vi "number to Boolean.vi"(1 "Numeric":dbl) -> (0 "Boolean":bool)   [LabVIEW 2023]
doc: "If input number (real or integer) is zero, outputs a \"false\". Otherwise, outputs a \"true\"."
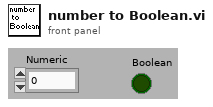
[diagram p1: front panel]
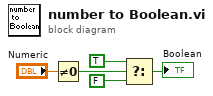
[diagram p0: block diagram]
diagram:
  n1 = Not Equal To 0?(x="Numeric") -> (x != 0?=w4:bool)
  n2 = Select(t=TRUE, s=w4, f=FALSE) -> (s? t:f=→"Boolean":bool)
